vi "Vision Processing.vi"(6 "LED Color":T5={"Hue"={23.67058792990901, 48.923317529462665}, "Sat"={66.78571428571429, 255.0}, "Val"={48.571428571428584, 255.0}} {"Hue" scale=0.0..255.0 scale format="%#_3g"}, 7 "Image Src":T1) -> (0 "Detected Targets":T2(array[cluster]) {"Normalized Rect"."Numeric 5" format="%#_2g"; "Normalized Rect"."Numeric 3" format="%#_2g"; "Normalized Rect"."Numeric 2" format="%#_2g"; "Normalized Rect"."Numeric" format="%#_2g"}, 1 "Sorted Particle Scores":T3(array[cluster]) {"Moment Factor" format="%#_3g"; "Aspect Ratio" format="%#_3g"; "Area to CH" format="%#_3g"; "X" format="%#_3g"; "Y" format="%#_3g"}, 2 "Masked":T1(plugin-control), 3 "Original Image":T1(plugin-control))   [LabVIEW 2015]
uses:
  Camera Types.ctl
  <vilib>/vision/Image Controls.llb/IMAQ Image.ctl
  <vilib>/vision/NI_Vision_Development_Module.lvlib
panel:
  out "Highest Avg Score":dbl
  in  "Min Score Threshold":i32=75
  in  "Display Original":bool=TRUE
  in  "Display Mask":bool=TRUE
  in  "Emphasize Limit Tests":bool=TRUE
  in  "Camera Type":T4=enum."MS HD3000 square"
  in  "Aspect Fudge Factor":dbl=1.0
  in  "Score Threshold":dbl=75.0
  out "Qualified Particles":i32
  # "Density Profile"
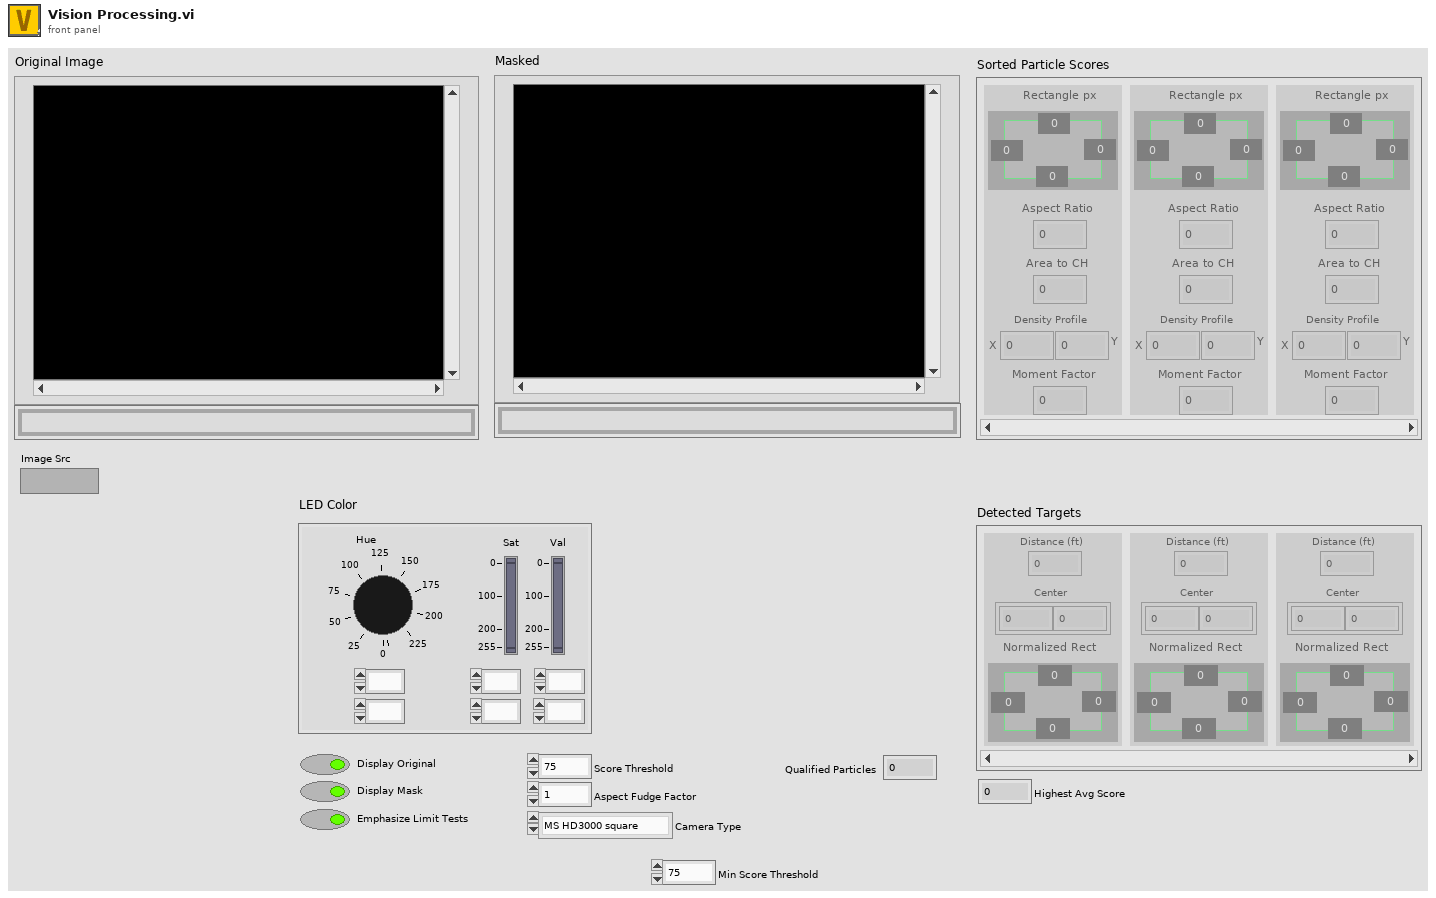
[diagram p1: front panel]
types:
  T1 = typedef "IMAQ Image.ctl" = refnum<image>
  T2 = cluster{"Distance (ft)":dbl, "Center":cluster{dbl, dbl}, "Normalized Rect":cluster{"Numeric":dbl, "Numeric 2":dbl, "Numeric 3":dbl, "Numeric 5":dbl}}[]
  T3 = cluster{"Rectangle px":cluster{"Numeric":dbl, "Numeric 2":dbl, "Numeric 3":dbl, "Numeric 5":dbl}, "Aspect Ratio":dbl, "Area to CH":dbl, "X":dbl, "Y":dbl, "Moment Factor":dbl}[]
  T4 = typedef "Camera Types.ctl" = enum16{"206", "1011", "1013", "MS HD3000 square", "MS HD3000 640x480"}
  T5 = cluster{"Hue":cluster{dbl, dbl}, "Sat":cluster{dbl, dbl}, "Val":cluster{dbl, dbl}}
  T6 = typedef "Particle Parameters" = i32
  T7 = typedef "Image Type" = u32
  T8 = cluster{"Bounding box":cluster{"left":dbl, "top":dbl, "right":dbl, "bottom":dbl}, "Aspect Ratio":dbl, "Area to CH":dbl, "X Mask":dbl, "Y Mask":dbl, "Moment":dbl}[]
  T9 = cluster{"Rectangle":cluster{"Numeric":dbl, "Numeric 2":dbl, "Numeric 3":dbl, "Numeric 5":dbl}, "L":dbl, "Area to CH":dbl, "X":dbl, "Y":dbl, "Moment Factor":dbl}[]
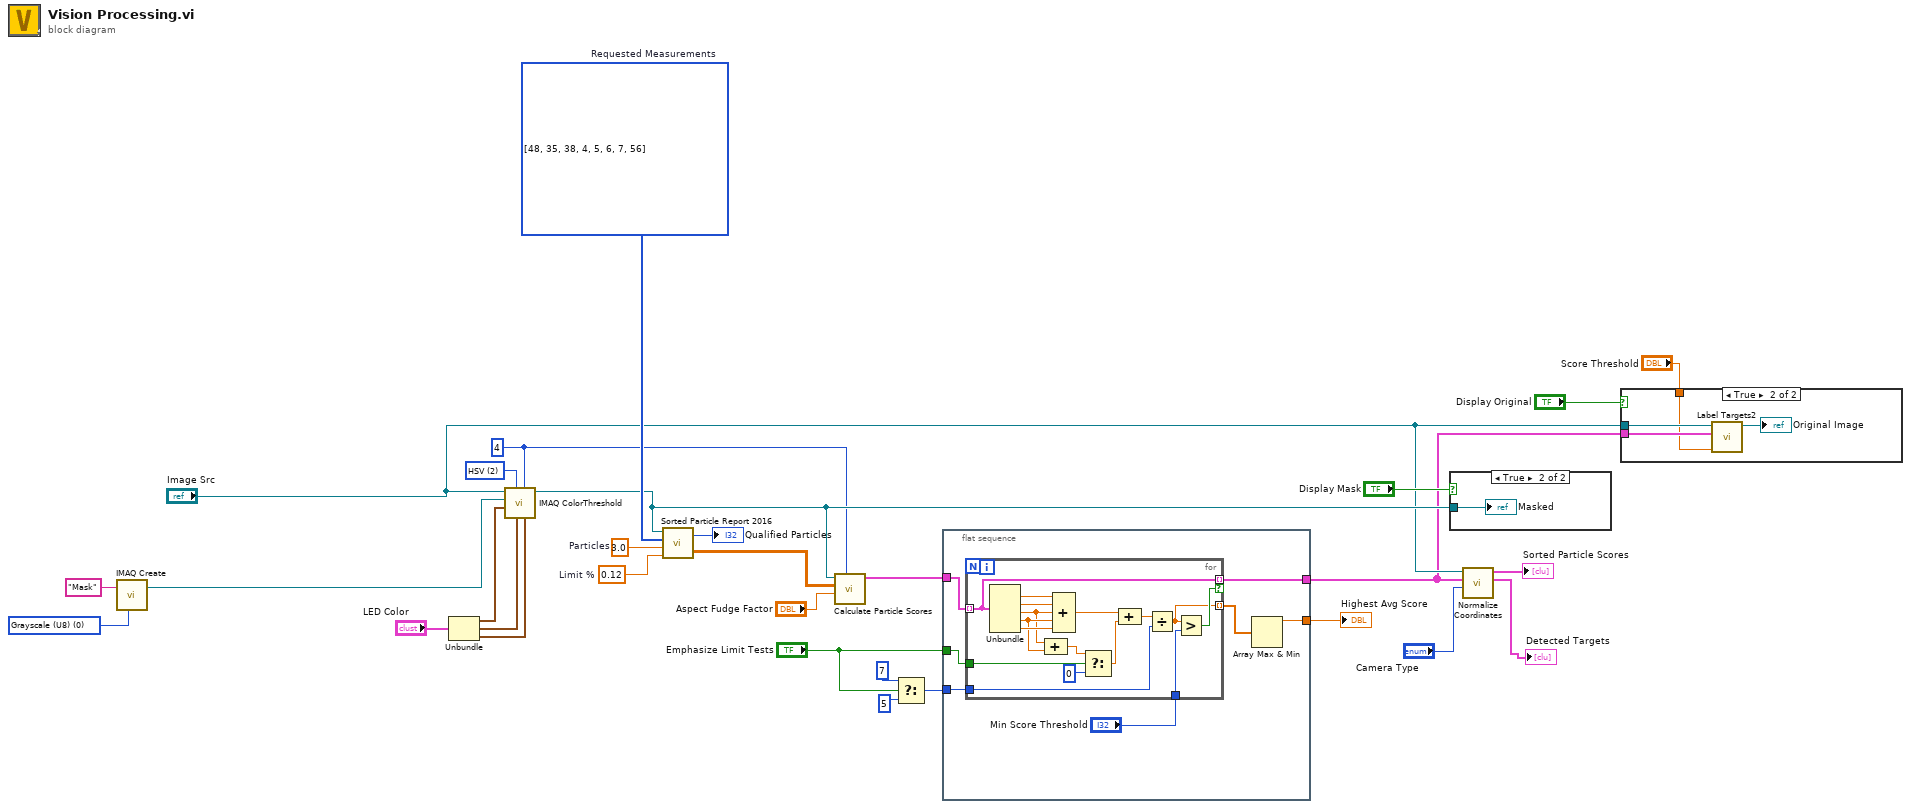
[diagram p0: block diagram]
diagram:
  w3 = 4 ("Replace Value")
  w17 = u16 2 items=["RGB", "HSL", "HSV", "HSI"] ("Color Mode")
  w20 = 0.12  # Limit %
  w22 = 3.0  # Particles
  w27 = T6[] [48, 35, 38, 4, 5, 6, 7, 56] items=["Center of Mass X", "Center of Mass Y", "First Pixel X", "First Pixel Y", "Bounding Rect Left", "Bounding Rect Top", "Bounding Rect Right", "Bounding Rect Bottom", "Max Feret Diameter Start X", "Max Feret Diameter Start Y", "Max Feret Diameter End X", "Max Feret Diameter End Y", "Max Horiz. Segment Length Left", "Max Horiz. Segment Length Right", "Max Horiz. Segment Length Row", "-", "Bounding Rect Width", "Bounding Rect Height", "Bounding Rect Diagonal", "Perimeter", "Convex Hull Perimeter", "Holes' Perimeter", "Max Feret Diameter", "Equivalent Ellipse Major Axis", "Equivalent Ellipse Minor Axis", "Equivalent Ellipse Minor Axis (Feret)", "Equivalent Rect Long Side", "Equivalent Rect Short Side", "Equivalent Rect Diagonal", "Equivalent Rect Short Side (Feret)", "Average Horiz. Segment Length", "Average Vert. Segment Length", "Hydraulic Radius", "Waddel Disk Diameter", "-", "Area", "Holes' Area", "Particle & Holes' Area", "Convex Hull Area", "Image Area", "-", "Number of Holes", "Number of Horiz. Segments", "Number of Vert. Segments", "-", "Orientation", "Max Feret Diameter Orientation", "-", "% Area/Image Area", "% Area/(Particle & Holes' Area)", "Ratio of Equivalent Ellipse Axes", "Ratio of Equivalent Rect Sides", "-", "Elongation Factor", "Compactness Factor", "Heywood Circularity Factor", "Type Factor", "-", "Sum X", "Sum Y", "Sum XX", "Sum XY", "Sum YY", "Sum XXX", "Sum XXY", "Sum XYY", "Sum YYY", "-", "Moment of Inertia XX", "Moment of Inertia XY", "Moment of Inertia YY", "Moment of Inertia XXX", "Moment of Inertia XXY", "Moment of Inertia XYY", "Moment of Inertia YYY", "Norm. Moment of Inertia XX", "Norm. Moment of Inertia XY", "Norm. Moment of Inertia YY", "Norm. Moment of Inertia XXX", "Norm. Moment of Inertia XXY", "Norm. Moment of Inertia XYY", "Norm. Moment of Inertia YYY", "Hu Moment 1", "Hu Moment 2", "Hu Moment 3", "Hu Moment 4", "Hu Moment 5", "Hu Moment 6", "Hu Moment 7"]  # Requested Measurements
  w30 = T7 0 items=["Grayscale (U8)", "Grayscale (I16)", "Grayscale (SGL)", "Complex (CSG)", "RGB (U32)", "HSL (U32)", "RGB (U64)", "Grayscale (U16)"] ("Image Type")
  n1 = call "IMAQ Create"("Image Name"="Mask", "Image Type"=w30) -> ("New Image"=w28:T1)  [unwired: 2 in, 2 out]
  n2 = Unbundle("LED Color") -> ("Hue"=w26:cluster{dbl, dbl}, "Sat"=w25:cluster{dbl, dbl}, "Val"=w24:cluster{dbl, dbl})
  n3 = call "IMAQ ColorThreshold"("Blue or Luma or Val or Inten Range"=w24, "Replace Value"=w3, "Green or Sat Range"=w25, "Color Mode"=w17, "Red or Hue Range"=w26, "Image Dst"=w28, "Image Src"="Image Src") -> ("Image Dst Out"=w16:T1)  [unwired: 3 in, 1 out]
  n4 = call "Sorted Particle Report 2016.vi"("Min Area Size %"=w20, "Particle Count Limit"=w22, "Pixel Measurements"=w27, "Image in"=w16) -> ("Sorted Data"=w15:dbl[][], "Particles"=→"Qualified Particles":i32)
  n5 = call "Calculate Particle Scores.vi"("Pixel Value"=w3, "Aspect Fudge Factor"="Aspect Fudge Factor", "Sorted Data"=w15, "Image in"=w16) -> ("Scores"=w13:T8)  [unwired: 7 in]
  n6 = Select(t=7, s="Emphasize Limit Tests", f=5) -> (s? t:f=w10:i32)
  n7 = flat-sequence {
    tunnel: w13 -> [w36]
    tunnel: w10 -> [w34]
    tunnel: [w37] -> w9
    tunnel: [w31] -> w5
    tunnel: "Emphasize Limit Tests" -> [w35]
    frame #0 {
      n8 = for {
        tunnel: w36 -> [w51] mode=indexing
        tunnel: [w51] -> w31 mode=indexing if=w50
        tunnel: [w49] -> w32 mode=indexing
        tunnel: w34 -> [w48]
        tunnel: "Min Score Threshold" -> [w47]
        tunnel: w35 -> [w40]
        n9 = Unbundle(w51) -> ("Aspect Ratio"=w53:dbl, "Area to CH"=w52:dbl, "X Mask"=w42:dbl, "Y Mask"=w43:dbl, "Moment"=w44:dbl)  [unwired: 1 out]
        n10 = Compound Arithmetic op=ADD(w42, w43) -> (w41:dbl)
        n11 = Compound Arithmetic op=ADD(w53, w52, w42, w43, w44) -> (w46:dbl)
        n12 = Select(t=w41, s=w40, f=0) -> (s? t:f=w39:dbl)
        n13 = Compound Arithmetic op=ADD(w46, w39) -> (w45:dbl)
        n14 = Divide(x=w45, y=w48) -> (x/y=w49:dbl)
        n15 = Greater?(x=w49, y=w47) -> (0:w50:bool)
      }
      n16 = Array Max & Min(array=w32) -> (max value=w37:dbl)  [unwired: 3 out]
    }
  }
  n17 = case shown="True" "Display Mask" {
    tunnel: w16 -> [_ w54]
    frame False {
    }
    frame True {
      "Masked" <- w54
    }
  }
  n18 = call "Normalize Coordinates.vi"("Camera Type"="Camera Type", "Targets"=w5, "Image in"="Image Src") -> ("Found Targets"=→"Detected Targets":T2, "Sorted Scores"=→"Sorted Particle Scores":T9)  [unwired: 7 in]
  n19 = case shown="True" "Display Original" {
    tunnel: "Image Src" -> [_ w58]
    tunnel: w5 -> [_ w56]
    tunnel: "Score Threshold" -> [_ w55]
    frame False {
    }
    frame True {
      n20 = call "Label Targets2.vi"("Score Threshold"=w55, "Targets"=w56, "Image in"=w58) -> ("Image out"=→"Original Image":T1)  [unwired: 8 in]
    }
  }
  "Highest Avg Score" <- w9
